vi "Updata CtrlStates.vi"(8 "error in (no error)":errorcluster caption="错误输入（无错误）", 10 "State":enum16{"Config", "Run", "Pause", "Stop", "Save"}(ring)=enum."Run", 11 "Ctrls*":refnum<vi>[](array[refnum])) -> (0 "error out":errorcluster caption="错误输出")   [LabVIEW 2016]
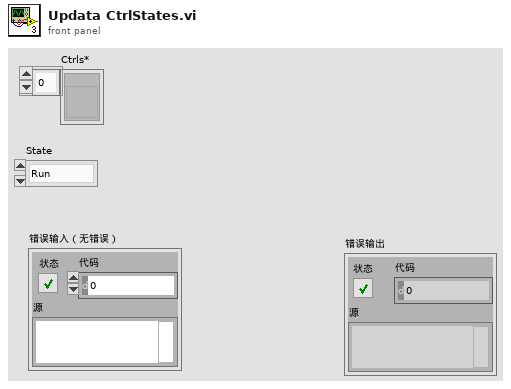
[diagram p1: front panel]
types:
  T1 = enum8{"Enabled", "Disabled", "Disabled and Grayed Out"}[]
  T2 = typedef "Global para Config.ctl" = cluster{"连续存储设置":cluster{"Save Mode":i32, "Sel Save Mode":i32, "FolderPath":path, "Filename":string, "Explation":string, "AutoPoint":i32, "Template":path}, "Latest Prj":path, "Tdms Ref*":refnum<k34>, "默认波形图个数":u8, "列表列数":u8}
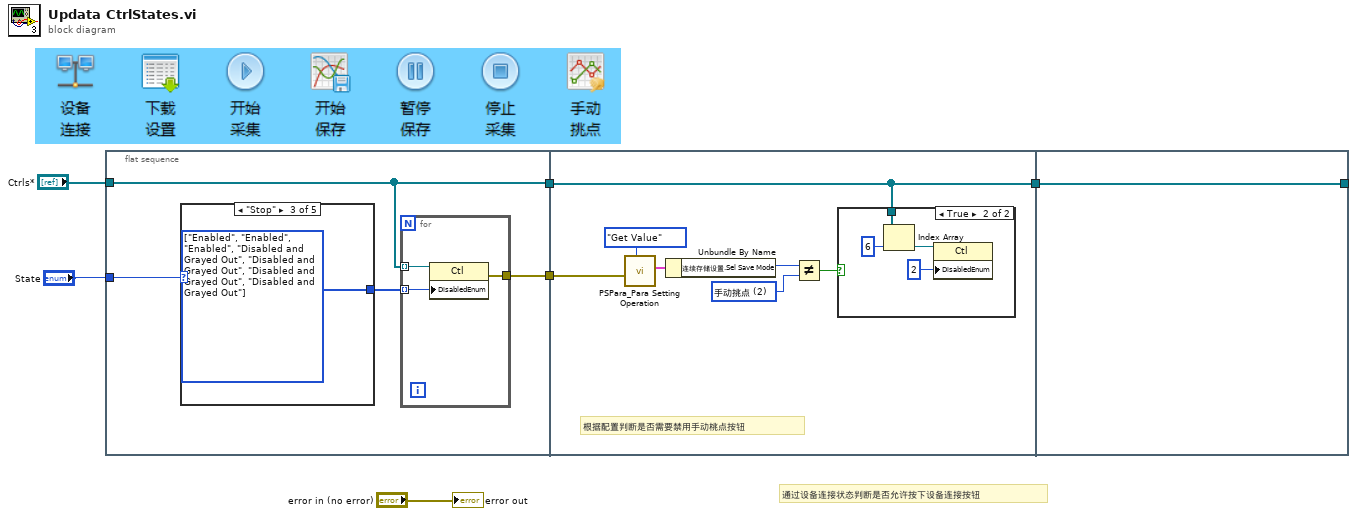
[diagram p0: block diagram]
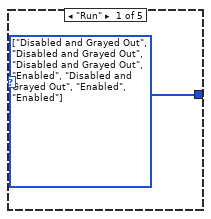
[diagram p2: hidden frame]
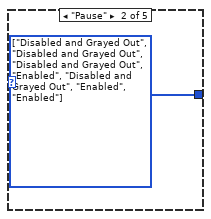
[diagram p3: hidden frame]
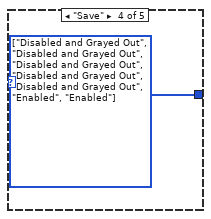
[diagram p4: hidden frame]
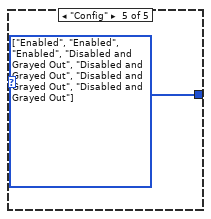
[diagram p5: hidden frame]
diagram:
  # "通过设备连接状态判断是否允许按下设备连接按钮"
  n1 = flat-sequence {
    tunnel: "State" -> [w10]
    tunnel: "Ctrls*" -> [w7]
    tunnel: [w8] -> w4
    tunnel: [w7] -> w3
    tunnel: w4 -> [w21]
    tunnel: w3 -> [w20]
    tunnel: [w20] -> w1
    tunnel: [w30] -> _
    tunnel: w1 -> [w30]
    frame #0 {
      n2 = case shown="\"Stop\"" w10 {
        tunnel: [w14 w15 w16 w17 w18] -> w9
        frame "Run" {
          w14 = T1 [enum."Disabled and Grayed Out", enum."Disabled and Grayed Out", enum."Disabled and Grayed Out", enum."Enabled", enum."Disabled and Grayed Out", enum."Enabled", enum."Enabled"] items=["Enabled", "Disabled", "Disabled and Grayed Out"]
        }
        frame "Pause" {
          w15 = T1 [enum."Disabled and Grayed Out", enum."Disabled and Grayed Out", enum."Disabled and Grayed Out", enum."Enabled", enum."Disabled and Grayed Out", enum."Enabled", enum."Enabled"] items=["Enabled", "Disabled", "Disabled and Grayed Out"]
        }
        frame "Stop" {
          w16 = T1 [enum."Enabled", enum."Enabled", enum."Enabled", enum."Disabled and Grayed Out", enum."Disabled and Grayed Out", enum."Disabled and Grayed Out", enum."Disabled and Grayed Out"] items=["Enabled", "Disabled", "Disabled and Grayed Out"]
        }
        frame "Save" {
          w17 = T1 [enum."Disabled and Grayed Out", enum."Disabled and Grayed Out", enum."Disabled and Grayed Out", enum."Disabled and Grayed Out", enum."Disabled and Grayed Out", enum."Enabled", enum."Enabled"] items=["Enabled", "Disabled", "Disabled and Grayed Out"]
        }
        frame "Config" {
          w18 = T1 [enum."Enabled", enum."Enabled", enum."Enabled", enum."Disabled and Grayed Out", enum."Disabled and Grayed Out", enum."Disabled and Grayed Out", enum."Disabled and Grayed Out"] items=["Enabled", "Disabled", "Disabled and Grayed Out"]
        }
      }
      n3 = for {
        tunnel: w7 -> [w13] mode=indexing
        tunnel: w9 -> [w12] mode=indexing
        tunnel: [w11] -> w8
        n4 = property class="Ctl"(reference=w13, "DisabledEnum"=w12) -> (error out=w11:errorcluster)  [unwired: 1 in, 1 out]
      }
    }
    frame #1 {
      w22 = 2 items=["不挑点", "自动挑点", "手动挑点"] ("Save Mode")
      # "根据配置判断是否需要禁用手动桃点按钮"
      n5 = call "PSPara_Para Setting Operation.vi"("Operation"=enum16{"Set Value", "Get Value", "Initialize"}."Get Value", "error in (no error)"=w21) -> ("_Para"=w24:T2)  [unwired: 8 in, 1 out]
      n6 = Unbundle By Name(w24) -> ("连续存储设置.Sel Save Mode"=w23:i32)
      n7 = Not Equal?(x=w23, y=w22) -> (x != y?=w19:bool)
      n8 = case shown="True" w19 {
        tunnel: w20 -> [_ w28]
        frame False {
        }
        frame True {
          n9 = Index Array(array=w28, index=6 ("索引")) -> (element=w29:refnum<vi>)
          n10 = property class="Ctl"(reference=w29, "DisabledEnum"=2 ("索引")) -> ()  [unwired: 1 in, 2 out]
        }
      }
    }
    frame #2 {
    }
  }
  "error out" <- "error in (no error)"
